vi "Ustalenie nowego przesunięcia mapy po mose down-up.vi"(7 "Właściwości mapy in":T5, 8 "Pocz. poł.":T1 {"UTM"."N [m]" format="%#_10g"}, 9 "Obsługa punktów in":T7, 10 "Mouse down \ncoords":T2, 11 "Mouse":T6) -> (2 "Właściwości mapy out":T4, 3 "Obsługa punktów out":T7)   [LabVIEW 2012, in "Biblioteka moduł map v3.lvlib" / "Pomocnicze.lvlib"]
doc: "Ustalenie nowego przesunięcia mapy na podstawie aktualnego położenia oraz różnicy pomiędzy położeniem kursorów po mouse up i po mouse down. Ustalane jest również położenie ostatnio zaznaczonego punktu."
uses:
  Pomocnicze.lvlib
  <vilib>/Utility/miscctls.llb/LVMouseTypeDef.ctl
  <vilib>/Utility/miscctls.llb/LVBoundsTypeDef.ctl
  <vilib>/Utility/miscctls.llb/LVPoint32TypeDef.ctl
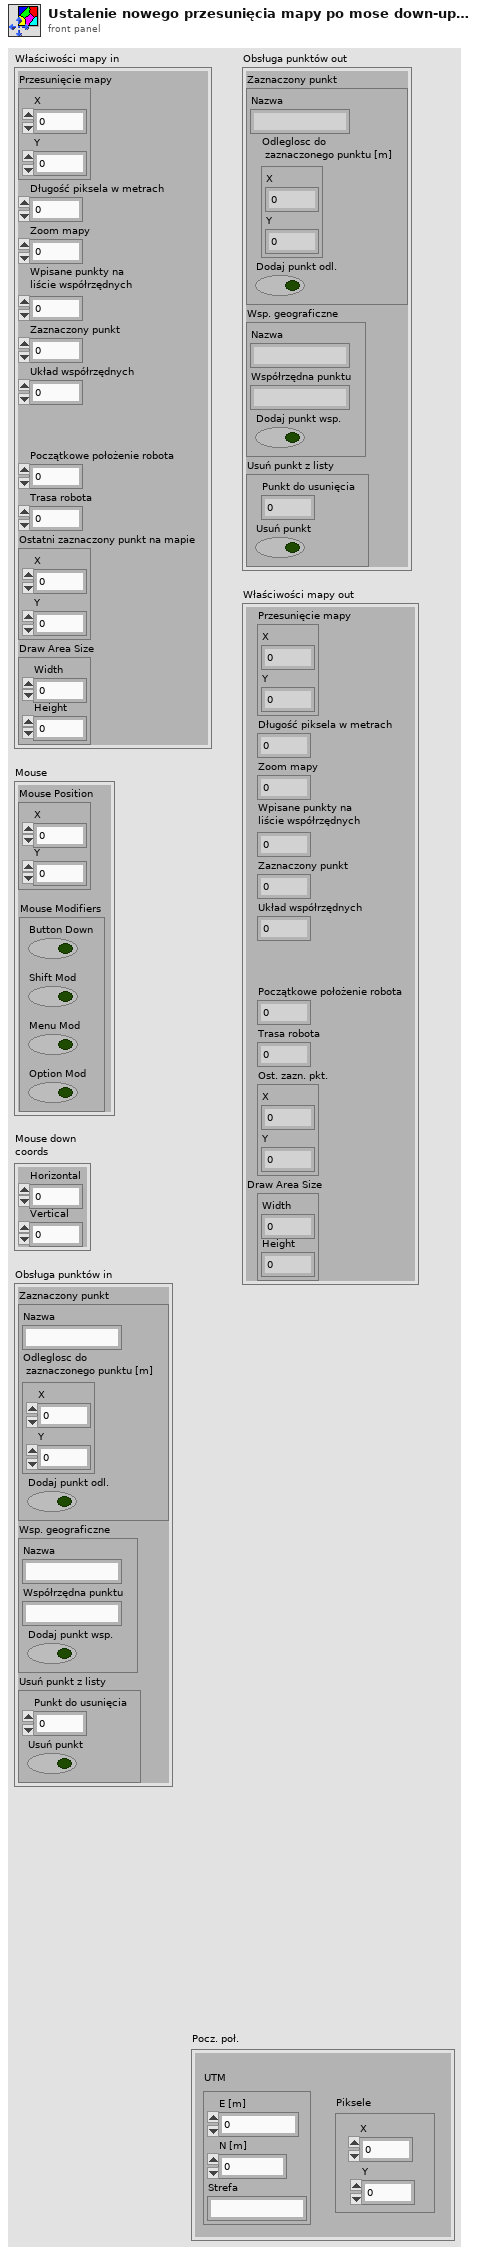
[diagram p1: front panel]
types:
  T1 = cluster{"UTM":cluster{"E [m]":ext, "N [m]":ext, "Strefa":string}, "Piksele":cluster{"X":i32, "Y":i32}}
  T2 = typedef "LVPoint32TypeDef.ctl" = cluster{"Horizontal":i32, "Vertical":i32}
  T3 = typedef "LVBoundsTypeDef.ctl" = cluster{"Width":u32, "Height":u32}
  T4 = cluster{"Przesunięcie mapy":cluster{"X":i16, "Y":i16}, "Długość piksela w metrach":dbl, "Zoom mapy":sgl, "Wpisane punkty na\nliście współrzędnych":u32, "Zaznaczony punkt":u32, "Układ współrzędnych":u32, "Początkowe położenie robota":u32, "Trasa robota":u32, "Ost. zazn. pkt.":cluster{"X":i32, "Y":i32}, "Draw Area Size":T3}
  T5 = cluster{"Przesunięcie mapy":cluster{"X":i16, "Y":i16}, "Długość piksela w metrach":dbl, "Zoom mapy":sgl, "Wpisane punkty na\nliście współrzędnych":u32, "Zaznaczony punkt":u32, "Układ współrzędnych":u32, "Początkowe położenie robota":u32, "Trasa robota":u32, "Ostatni zaznaczony punkt na mapie":cluster{"X":i32, "Y":i32}, "Draw Area Size":T3}
  T6 = typedef "LVMouseTypeDef.ctl" = cluster{"Mouse Position":cluster{"X":i32, "Y":i32}, "Mouse Modifiers":cluster{"Button Down":bool, "Shift Mod":bool, "Menu Mod":bool, "Option Mod":bool}}
  T7 = cluster{"Zaznaczony punkt":cluster{"Nazwa":string, "Odleglosc do\n zaznaczonego punktu [m]":cluster{"X":dbl, "Y":dbl}, "Dodaj punkt odl.":bool}, "Wsp. geograficzne":cluster{"Nazwa":string, "Współrzędna punktu":string, "Dodaj punkt wsp.":bool}, "Usuń punkt z listy":cluster{"Punkt do usunięcia":u16, "Usuń punkt":bool}}
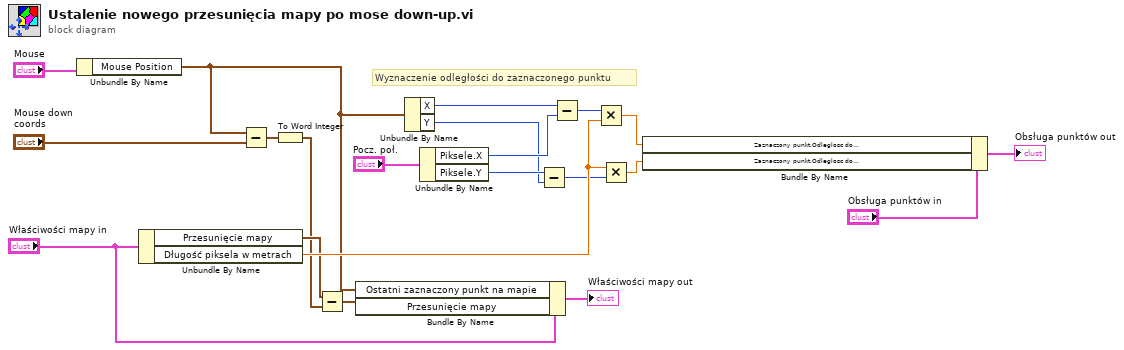
[diagram p0: block diagram]
diagram:
  # "Wyznaczenie odległości do zaznaczonego punktu"
  n1 = Unbundle By Name("Mouse") -> ("Mouse Position"=w4:cluster{"X":i32, "Y":i32})
  n2 = Unbundle By Name("Właściwości mapy in") -> ("Przesunięcie mapy"=w6:cluster{"X":i16, "Y":i16}, "Długość piksela w metrach"=w17:dbl)
  n3 = Subtract(x=w4, y="Mouse down \ncoords") -> (x-y=w2:T2)
  n4 = To Word Integer(number=w2) -> (16bit integer=w1:cluster{"Horizontal":i16, "Vertical":i16})
  n5 = Subtract(x=w6, y=w1) -> (x-y=w5:cluster{i16, i16})
  n6 = Bundle By Name(cluster="Właściwości mapy in", "Ostatni zaznaczony punkt na mapie"=w4, "Przesunięcie mapy"=w5) -> (→"Właściwości mapy out":T5)
  n7 = Unbundle By Name(w4) -> ("X"=w8:i32, "Y"=w9:i32)
  n8 = Unbundle By Name("Pocz. poł.") -> ("Piksele.X"=w13:i32, "Piksele.Y"=w14:i32)
  n9 = Subtract(x=w14, y=w9) -> (x-y=w10:i32)
  n10 = Subtract(x=w8, y=w13) -> (x-y=w16:i32)
  n11 = Multiply(x=w16, y=w17) -> (x*y=w19:dbl)
  n12 = Multiply(x=w17, y=w10) -> (x*y=w20:dbl)
  n13 = Bundle By Name(cluster="Obsługa punktów in", "Zaznaczony punkt.Odleglosc do\n zaznaczonego punktu [m].X"=w19, "Zaznaczony punkt.Odleglosc do\n zaznaczonego punktu [m].Y"=w20) -> (→"Obsługa punktów out":T7)
